vi "Wait for Operation Complete.vi"(8 "error in (no error)":errorcluster, 10 "Maximum Time (10000 ms)":i32=10000 min=0, 11 "VISA session":refnum<visa-resource-name>) -> (0 "error out":errorcluster, 3 "dup VISA session":refnum<visa-resource-name>)   [LabVIEW 2013, in "Fluke 5XXX Series Multicalibrators.lvlib"]
doc: "This VI prevents other VIs from being executed before the calibrator has finished its current operation. This is useful for VIs that need to finish before subsequent VIs can run, such as waiting for a voltage to settle."
uses:
  Fluke 5XXX Series Multicalibrators.lvlib
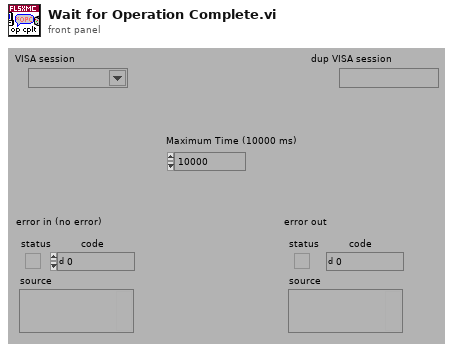
[diagram p1: front panel]
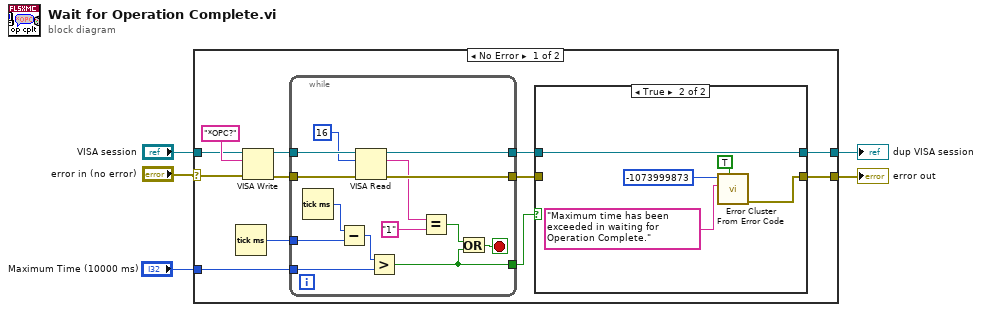
[diagram p0: block diagram]
diagram:
  n1 = case shown="No Error" "error in (no error)" {
    selector: "error in (no error)" -> [w13 w39]
    tunnel: "VISA session" -> [w16 w40]
    tunnel: [w8 w40] -> w4
    tunnel: [w6 w39] -> w3
    tunnel: "Maximum Time (10000 ms)" -> [w12 _]
    frame No Error {
      n2 = Tick Count (ms)() -> (millisecond timer value=w11:u32)
      n3 = VISA Write(VISA resource name=w16, write buffer="*OPC?" ("Reset Command"), error in (no error)=w13) -> (VISA resource name out=w15:refnum<visa-resource-name>, error out=w14:errorcluster)  [unwired: 1 out]
      n4 = while {
        tunnel: w15 -> [w38]
        tunnel: w14 -> [w37]
        tunnel: [w35] -> w7
        tunnel: [w34] -> w9
        tunnel: w12 -> [w26]
        tunnel: w11 -> [w28]
        tunnel: [w25] -> w10
        stop <- w30 stop-if-true
        n5 = Tick Count (ms)() -> (millisecond timer value=w29:u32)
        n6 = Subtract(x=w29, y=w28) -> (x-y=w27:u32)
        n7 = VISA Read(VISA resource name=w38, byte count=u32 16, error in (no error)=w37) -> (VISA resource name out=w34:refnum<visa-resource-name>, read buffer=w32:string, error out=w35:errorcluster)  [unwired: 1 out]
        n8 = Greater?(x=w27, y=w26) -> (0:w25:bool)
        n9 = Equal?(x=w32, y="1" ("x")) -> (x = y?=w31:bool)
        n10 = Or(x=w31, y=w25) -> (x .or. y?=w30:bool)
      }
      n11 = case shown="True" w10 {
        tunnel: w9 -> [w19 w24]
        tunnel: [w19 w24] -> w8
        tunnel: w7 -> [w18 _]
        tunnel: [w18 w23] -> w6
        frame False {
        }
        frame True {
          n12 = call <vilib>:"Error Cluster From Error Code.vi"("show call chain? (False)"=TRUE, "error message (\"\")"="Maximum time has been exceeded in waiting for Operation Complete." ("source"), "error code (0)"=-1073999873 ("code")) -> ("error out"=w23:errorcluster)  [unwired: 6 in]
        }
      }
    }
    frame Error {
    }
  }
  "dup VISA session" <- w4
  "error out" <- w3
